vi "oa_SCL Draw Cartesian Axes.vi"(5 "[user-specified font]":T3, 7 "desired font(Application)":T2(ring)=enum."Application Font", 8 "grid cosmetics":T1={"line color"=39168, "text color"=65280, "tick length(3)"=3, "crossing axes"=FALSE, "visible grid?"=TRUE}, 9 "axis attributes":T5={"x minimum"=0.0, "x maximum"=0.0, "x log?"=FALSE, "x precision"=1, "x format"=enum."Decimal", "y minimum"=0.0, "y maximum"=0.0, "y log?"=FALSE, "y precision"=1, "y format"=enum."Decimal"} {"x minimum" format="%0.2f"; "x maximum" format="%0.2f"; "y minimum" format="%0.2f"; "y maximum" format="%0.2f"}, 10 "bounding rect":T4, 11 "picture":picture) -> (1 "y scale factors":cluster{"a":dbl, "b":dbl, "log?":bool} {"b" format="%0.2f"; "a" format="%0.2f"}, 2 "x scale factors":cluster{"a":dbl, "b":dbl, "log?":bool} {"b" format="%0.2f"; "a" format="%0.2f"}, 3 "new picture":picture)   [LabVIEW 2017]
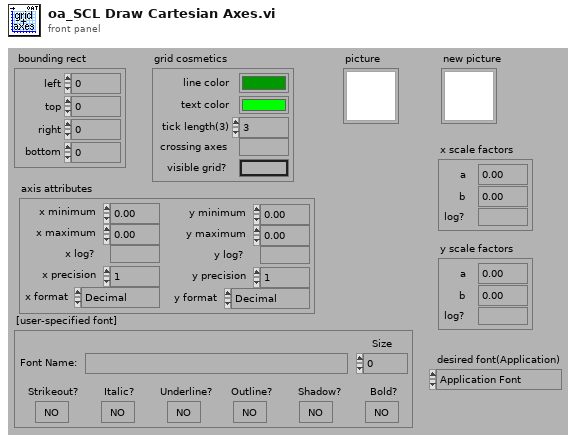
[diagram p1: front panel]
types:
  T1 = cluster{"line color":u32, "text color":u32, "tick length(3)":i16, "crossing axes":bool, "visible grid?":bool}
  T2 = enum16{"User-specified Font", "Application Font", "System Font", "Dialog Font"}
  T3 = cluster{"Font Name:":string, "Size":i16, "Strikeout?":bool, "Italic?":bool, "Underline?":bool, "Outline?":bool, "Shadow?":bool, "Bold?":bool}
  T4 = cluster{"left":i16, "top":i16, "right":i16, "bottom":i16}
  T5 = cluster{"x minimum":dbl, "x maximum":dbl, "x log?":bool, "x precision":u8, "x format":enum8{"Decimal", "Scientific", "Engineering", "Binary", "Octal", "Hex"}, "y minimum":dbl, "y maximum":dbl, "y log?":bool, "y precision":u8, "y format":enum8{"Decimal", "Scientific", "Engineering", "Binary", "Octal", "Hex"}}
  T6 = cluster{"coordinate 1":i16, "value 1":dbl, "coordinate 2":i16, "value 2":dbl, "log?":bool, "fmt and prec":cluster{"format":enum8{"Decimal", "Scientific", "Engineering", "Binary", "Octal", "Hex"}, "precision":u8}}
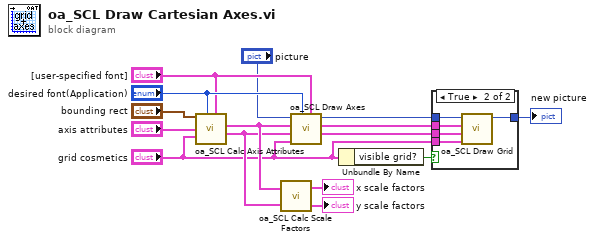
[diagram p0: block diagram]
diagram:
  n1 = call <vilib>:"oa_SCL Calc Axis Attributes.vi"("rect"="bounding rect", "desired font(Application)"="desired font(Application)", "xy axis"="axis attributes", "grid cosmetics"="grid cosmetics", "[user-specified font]"="[user-specified font]") -> ("x axis attributes"=w7:T6, "y axis attributes"=w6:T6)  [unwired: 4 in]
  n2 = call <vilib>:"oa_SCL Calc Scale Factors.vi"("y axis attributes"=w6, "x axis attributes"=w7) -> ("y scale factors"=→"y scale factors":cluster{"a":dbl, "b":dbl, "log?":bool}, "x scale factors"=→"x scale factors":cluster{"a":dbl, "b":dbl, "log?":bool})
  n3 = call <vilib>:"oa_SCL Draw Axes.vi"("[user-specified font]"="[user-specified font]", "desired font(Application)"="desired font(Application)", "grid cosmetics"="grid cosmetics", "y axis attributes"=w6, "x axis attributes"=w7, "picture"="picture") -> ("y scale specs"=w12:cluster{"coordinate":i16, "label":string}[], "x scale specs"=w13:cluster{"coordinate":i16, "label":string}[], "new picture"=w14:picture)  [unwired: 3 in]
  n4 = Unbundle By Name("grid cosmetics") -> ("visible grid?"=w11:bool)
  n5 = case shown="True" w11 {
    tunnel: w14 -> [w16 w21]
    tunnel: [w16 w20] -> w8
    tunnel: w13 -> [_ w19]
    tunnel: w12 -> [_ w18]
    tunnel: "grid cosmetics" -> [_ w17]
    frame False {
    }
    frame True {
      n6 = call <vilib>:"oa_SCL Draw Grid.vi"("grid cosmetics"=w17, "y scale specs"=w18, "x scale specs"=w19, "picture"=w21) -> ("new picture"=w20:picture)  [unwired: 7 in]
    }
  }
  "new picture" <- w8
